vi "Configure Resistor Band Visibility.vi"(8 "error in (no error)":errorcluster, 10 "Number of Bands in":u8, 11 "Color Box Refnum":refnum<vi>[](array[refnum])) -> (0 "error out":errorcluster, 2 "Number of Band out":u8)   [LabVIEW 2018, in "Front Panel Inteface.lvlib"]
uses:
  Front Panel Inteface.lvlib
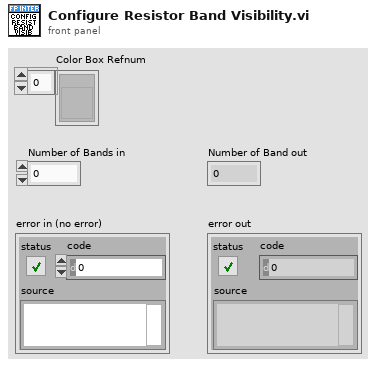
[diagram p1: front panel]
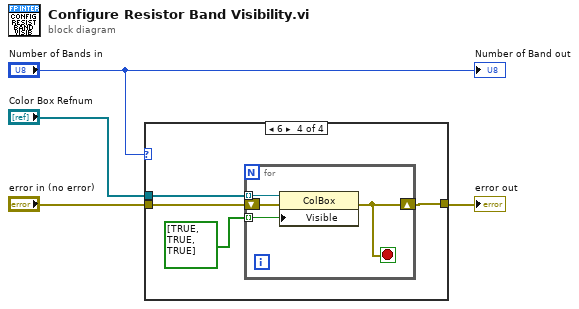
[diagram p0: block diagram]
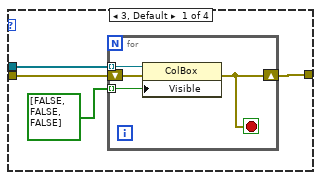
[diagram p2: hidden frame]
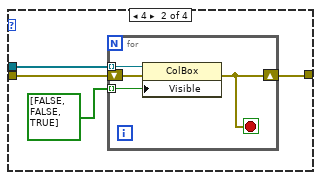
[diagram p3: hidden frame]
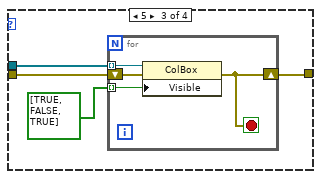
[diagram p4: hidden frame]
diagram:
  n1 = case shown="6" "Number of Bands in" {
    tunnel: "Color Box Refnum" -> [w5 w13 w23 w31]
    tunnel: "error in (no error)" -> [w7 w16 w22 w29]
    tunnel: [w6 w15 w21 w30] -> w1
    frame 3, Default {
      n2 = for {
        shift-right: [w11] -> w6
        shift-left: w7 -> [w12]
        tunnel: bool[] [FALSE, FALSE, FALSE] -> [w9] mode=indexing
        tunnel: w5 -> [w10] mode=indexing
        stop <- w11 stop-if-true
        n3 = property class="ColBox"(reference=w10, error in=w12, "Visible"=w9) -> (error out=w11:errorcluster)  [unwired: 1 out]
      }
    }
    frame 4 {
      n4 = for {
        shift-right: [w19] -> w15
        shift-left: w16 -> [w20]
        tunnel: bool[] [FALSE, FALSE, TRUE] -> [w17] mode=indexing
        tunnel: w13 -> [w18] mode=indexing
        stop <- w19 stop-if-true
        n5 = property class="ColBox"(reference=w18, error in=w20, "Visible"=w17) -> (error out=w19:errorcluster)  [unwired: 1 out]
      }
    }
    frame 5 {
      n6 = for {
        shift-right: [w27] -> w21
        shift-left: w22 -> [w28]
        tunnel: bool[] [TRUE, FALSE, TRUE] -> [w25] mode=indexing
        tunnel: w23 -> [w26] mode=indexing
        stop <- w27 stop-if-true
        n7 = property class="ColBox"(reference=w26, error in=w28, "Visible"=w25) -> (error out=w27:errorcluster)  [unwired: 1 out]
      }
    }
    frame 6 {
      n8 = for {
        shift-right: [w35] -> w30
        shift-left: w29 -> [w36]
        tunnel: bool[] [TRUE, TRUE, TRUE] -> [w33] mode=indexing
        tunnel: w31 -> [w34] mode=indexing
        stop <- w35 stop-if-true
        n9 = property class="ColBox"(reference=w34, error in=w36, "Visible"=w33) -> (error out=w35:errorcluster)  [unwired: 1 out]
      }
    }
  }
  "error out" <- w1
  "Number of Band out" <- "Number of Bands in"
